vi "Deadzone Limit.vi"(10 "Limit":dbl format="%#_13g", 11 "Input":dbl format="%#_13g") -> (3 "Output":dbl format="%#_13g")   [LabVIEW 2014]
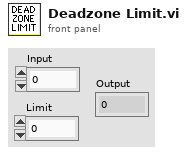
[diagram p1: front panel]
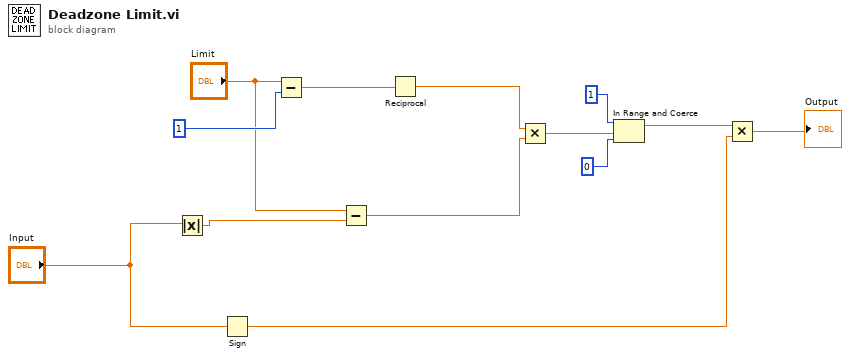
[diagram p0: block diagram]
diagram:
  n1 = Absolute Value(x="Input") -> (abs(x)=w2:dbl)
  n2 = Sign(1:"Input") -> (0:w1:dbl)
  n3 = Subtract(x="Limit", y=1) -> (x-y=w12:dbl)
  n4 = Subtract(x="Limit", y=w2) -> (x-y=w8:dbl)
  n5 = Reciprocal(x=w12) -> (1/x=w9:dbl)
  n6 = Multiply(x=w9, y=w8) -> (x*y=w7:dbl)
  n7 = In Range and Coerce(upper limit=1, x=w7, lower limit=0) -> (coerced(x)=w4:dbl)  [unwired: 1 out]
  n8 = Multiply(x=w4, y=w1) -> (x*y=→"Output":dbl)
